vi "Retrieve Side and Distance.vi"() -> (0 "Side":dbl, 1 "Distance (ft.)":dbl)   [LabVIEW 2013]
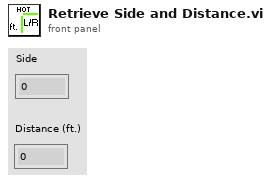
[diagram p1: front panel]
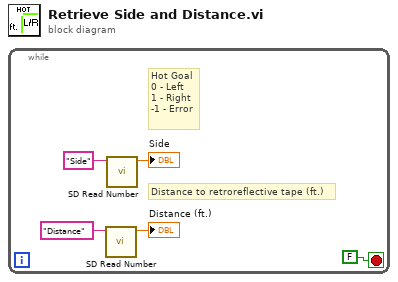
[diagram p0: block diagram]
diagram:
  n1 = while {
    stop <- FALSE stop-if-true
    # "Distance to retroreflective tape (ft.)"
    # "Hot Goal\n0 - Left\n1 - Right\n-1 - Error"
    n2 = call <vilib>:"SD Read Number.vi"("Name"="Distance") -> ("Numeric"=→"Distance (ft.)":dbl)  [unwired: 8 in, 2 out]
    n3 = call <vilib>:"SD Read Number.vi"("Name"="Side") -> ("Numeric"=→"Side":dbl)  [unwired: 8 in, 2 out]
  }
